vi "Analyzer.ReqFinder.vi"(10 "return value from python":string[](array[string]), 11 "Requirement to look":string) -> (3 "Req not found":bool)   [LabVIEW 2022 SP3, in "Analyzer.lvclass"]
uses:
  Analyzer.lvclass
  Analyzer.lvclass/Analyzer.ctl
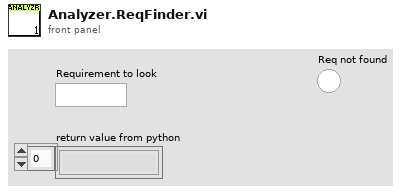
[diagram p1: front panel]
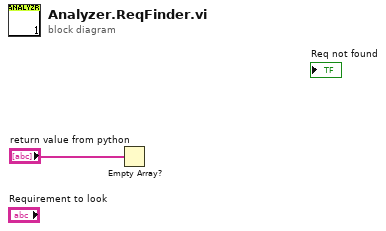
[diagram p0: block diagram]
diagram:
  n1 = Empty Array?(array="return value from python") -> ()  [unwired: 1 out]
